vi "Actor Core.vi"(8 "error in":errorcluster, 11 "Nested in":refnum<class "Thermometer Multichannel Worker.lvclass">) -> (0 "error out":errorcluster, 3 "Actor out":refnum<class "Actor.lvclass">)   [LabVIEW 2024, in "Thermometer Multichannel Worker.lvlib" / "Thermometer Multichannel Worker.lvclass"]
doc: "(<B>Filename</B>: Actor Framework.lvlib:Actor.lvclass:Actor Core.vi)\n\nReceives messages to the actor, reacts to them, and initiates any error handling that may shut the actor down.\n\nDescendant classes may override this VI to append parallel tasks for the actor to complete while it handles messages. Overrides use the Call Parent Method node."
uses:
  Thermometer Multichannel Worker.lvclass
  Thermometer Multichannel Worker.lvclass/Thermometer Multichannel Worker.ctl
  <vilib>/ActorFramework/Actor/Actor.lvclass
  <vilib>/ActorFramework/Stop Msg/Stop Msg.lvclass
  Thermometer Multichannel Worker Messages/Read Temperatures Msg/Read Temperatures Msg.lvclass
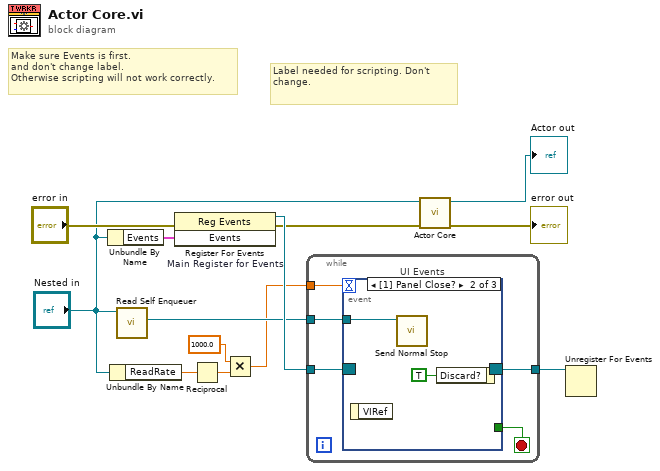
[diagram p0: block diagram]
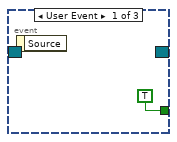
[diagram p2: hidden frame]
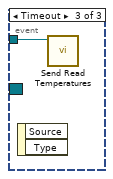
[diagram p3: hidden frame]
diagram:
  # "Label needed for scripting. Don't change."
  # "Make sure Events is first.\nand don't change label.\nOtherwise scripting will not work correctly."
  n1 = Unbundle By Name("Nested in") -> ("Events"=w10:cluster{"Stop":refnum<user-event>})
  n2 = Unbundle By Name("Nested in") -> ("ReadRate"=w3:dbl)
  n3 = call <vilib>:"Read Self Enqueuer.vi"("Actor"="Nested in") -> ("Self Enqueuer"=w8:refnum<class "Message Enqueuer.lvclass">)  [unwired: 10 in]
  n4 = register-events "Main Register for Events"(error in="error in", w10) -> (reference out=w11:refnum<event-registration>, error out=w6:errorcluster)  [unwired: 1 in]
  n5 = Reciprocal(x=w3) -> (1/x=w4:dbl)
  n6 = Multiply(x=1000.0, y=w4) -> (x*y=w2:dbl)
  n7 = while {
    tunnel: w11 -> [w18]
    tunnel: [w16] -> w9
    tunnel: w8 -> [w15]
    tunnel: w2 -> [w14]
    stop <- w17 stop-if-true
    n8 = event "UI Events" shown="[1] Panel Close?" {
      selector: w18 -> [_ _ _]
      dyn-events: [_ _ _] -> w16
      timeout: w14 -> [_ _ _]
      tunnel: [TRUE _ _] -> w17
      tunnel: w15 -> [_ w20 w22]
      event User Event {
        n9 = event-data() -> ()  [unwired: 1 in, 1 out]
      }
      event Panel Close? {
        n10 = event-data() -> ()  [unwired: 1 in, 1 out]
        n11 = call <vilib>:"Send Normal Stop.vi"("Message Enqueuer"=w20) -> ()  [unwired: 10 in, 1 out]
        n12 = event-data("Discard?"=TRUE) -> ()  [unwired: 1 in, 1 out]
      }
      event Timeout {
        n13 = event-data() -> ()  [unwired: 1 in, 2 out]
        n14 = call "Send Read Temperatures.vi"("Message Enqueuer"=w22) -> ()  [unwired: 9 in, 2 out]
      }
    }
  }
  n15 = call-parent "Actor Core.vi"("error in"=w6, "Actor in"="Nested in") -> ("error out"=→"error out":errorcluster, "Actor out"=→"Actor out":refnum<class "Actor.lvclass">)  [unwired: 8 in]
  n16 = Unregister For Events(event registration refnum=w9) -> ()  [unwired: 1 in, 1 out]
